vi "Read Analog Input.vi"(7 "ADC":i32, 8 "error in (no error)":errorcluster, 11 "VISA resource name in":refnum<visa-resource-name>) -> (0 "error out":errorcluster, 1 "Value":u16, 3 "VISA resource name":refnum<visa-resource-name>)   [LabVIEW 2024, in "CTIPicoVISA.lvlib"]
uses:
  CTIPicoVISA.lvlib
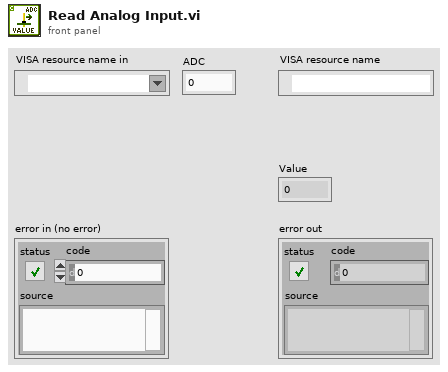
[diagram p1: front panel]
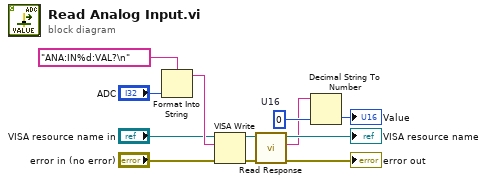
[diagram p0: block diagram]
diagram:
  w10 = u16 0  # U16
  n1 = Format Into String(format string="ANA:IN%d:VAL?\n", "ADC") -> (resulting string=w11:string)  [unwired: 2 in, 1 out]
  n2 = VISA Write(VISA resource name="VISA resource name in", write buffer=w11, error in (no error)="error in (no error)") -> (VISA resource name out=w5:refnum<visa-resource-name>, error out=w1:errorcluster)  [unwired: 1 out]
  n3 = call "Read Response.vi"("error in (no error)"=w1, "VISA resource name"=w5) -> ("error out"=→"error out":errorcluster, "Response"=w3:string, "VISA resource name Out"=→"VISA resource name":refnum<visa-resource-name>)  [unwired: 6 in, 1 out]
  n4 = Decimal String To Number(string=w3, default (0L)=w10) -> (number=→"Value":u16)  [unwired: 1 in, 1 out]
